vi "Generate Service Config JSON.vi"(0 "display name":string, 1 "description URL":string, 5 "service class":string, 7 "provided interfaces":string[](array[string]), 9 "path":string, 11 "error in":errorcluster, 12 "annotations":T1[](array[typedef])) -> (4 "service config JSON":string, 15 "error out":errorcluster)   [LabVIEW 2020, in "MeasurementLink Measurement Server.lvlib"]
uses:
  MeasurementLink Measurement Server.lvlib
  TypeDefs/Measurement Annotation.ctl
  867c5996-9fc4-446f-bc7e-cd1af3184270.vi
  b2866af8-bc70-4c0d-b595-9f5224cfa858.vi
  0c37daab-07df-4eb5-bca5-1a967d50c5e0.vi
  867c5996-9fc4-446f-bc7e-cd1af3184270.vi/49d2641b-58d2-418d-86ef-5c98235809e6.vi
  867c5996-9fc4-446f-bc7e-cd1af3184270.vi/729eb87d-9ab4-481c-bd0a-7090d6acb718.vi
  b2866af8-bc70-4c0d-b595-9f5224cfa858.vi/49d2641b-58d2-418d-86ef-5c98235809e6.vi
  b2866af8-bc70-4c0d-b595-9f5224cfa858.vi/729eb87d-9ab4-481c-bd0a-7090d6acb718.vi
  0c37daab-07df-4eb5-bca5-1a967d50c5e0.vi/49d2641b-58d2-418d-86ef-5c98235809e6.vi
  0c37daab-07df-4eb5-bca5-1a967d50c5e0.vi/729eb87d-9ab4-481c-bd0a-7090d6acb718.vi
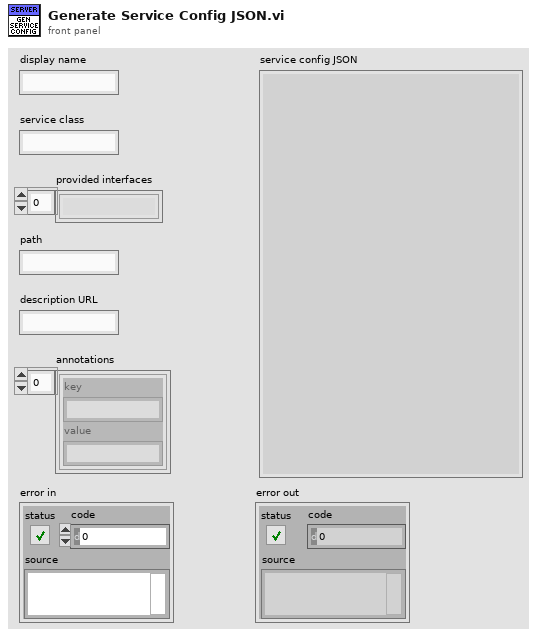
[diagram p1: front panel]
types:
  T1 = typedef "MeasurementLink Measurement Server.lvlib/Measurement Annotation.ctl" = cluster{"key":string, "value":string}
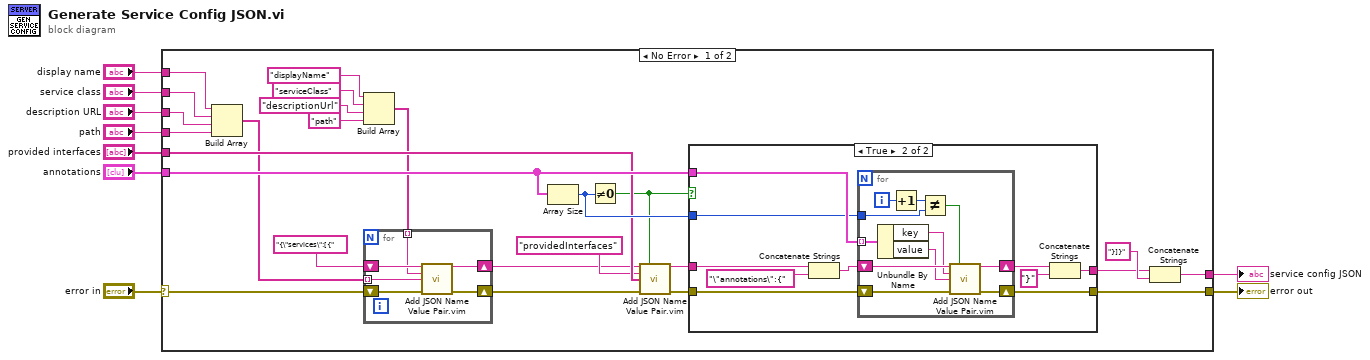
[diagram p0: block diagram]
diagram:
  n1 = case shown="No Error" "error in" {
    selector: "error in" -> [w28 w64]
    tunnel: [w32 w64] -> w8
    tunnel: "display name" -> [w21 _]
    tunnel: "service class" -> [w20 _]
    tunnel: "description URL" -> [w19 _]
    tunnel: [w33 _] -> w5
    tunnel: "path" -> [w18 _]
    tunnel: "provided interfaces" -> [w25 _]
    tunnel: "annotations" -> [w31 _]
    frame No Error {
      n2 = Build Array(w21, w20, w19, w18) -> (w15:string[])
      n3 = Build Array("displayName", "serviceClass", "descriptionUrl", "path") -> (w10:string[])
      n4 = for {
        shift-right: [w38] -> w17
        shift-left: w28 -> [w40]
        shift-right: [w37] -> w16
        shift-left: "{\"services\":[{" -> [w39]
        tunnel: w15 -> [w36] mode=indexing
        tunnel: w10 -> [w35] mode=indexing
        n5 = call "Add JSON Name Value Pair.vim"("JSON string in"=w39, "name"=w35, "value"=w36, "error in"=w40) -> ("JSON string out"=w37:string, "error out"=w38:errorcluster)  [unwired: 10 in]
      }
      n6 = Array Size(array=w31) -> (size(s)=w30:i32)
      n7 = Not Equal To 0?(x=w30) -> (x != 0?=w24:bool)
      n8 = call "Add JSON Name Value Pair.vim"("JSON string in"=w16, "include trailing comma"=w24, "name"="providedInterfaces", "value"=w25, "error in"=w17) -> ("JSON string out"=w23:string, "error out"=w26:errorcluster)  [unwired: 9 in]
      n9 = case shown="True" w24 {
        tunnel: w26 -> [w42 w52]
        tunnel: [w42 w51] -> w32
        tunnel: w31 -> [_ w50]
        tunnel: w30 -> [_ w47]
        tunnel: [w41 w44] -> w29
        tunnel: w23 -> [w41 w43]
        frame False {
        }
        frame True {
          n10 = Concatenate Strings(w43, "\"annotations\":{") -> (w48:string)
          n11 = for {
            shift-right: [w58] -> w51
            shift-left: w52 -> [w59]
            tunnel: w50 -> [w61] mode=indexing
            shift-right: [w56] -> w46
            shift-left: w48 -> [w57]
            tunnel: w47 -> [w60]
            i -> [w63]
            n12 = Unbundle By Name(w61) -> ("key"=w53:string, "value"=w54:string)
            n13 = Increment(x=w63) -> (x+1=w62:i32)
            n14 = Not Equal?(x=w62, y=w60) -> (x != y?=w55:bool)
            n15 = call "Add JSON Name Value Pair.vim"("JSON string in"=w57, "include trailing comma"=w55, "name"=w53, "value"=w54, "error in"=w59) -> ("JSON string out"=w56:string, "error out"=w58:errorcluster)  [unwired: 9 in]
          }
          n16 = Concatenate Strings(w46, "}") -> (w44:string)
        }
      }
      n17 = Concatenate Strings(w29, "}]}") -> (w33:string)
    }
    frame Error {
    }
  }
  "error out" <- w8
  "service config JSON" <- w5
